vi "MOVE FRAME.vi"(8 "error in (no error)":errorcluster, 9 "return value":cluster{"x":dbl, "y":dbl}, 10 "Boolean":bool, 11 "Queue in":refnum<queue>) -> (0 "error out":errorcluster, 1 "Initial coordinates (m)":cluster{"Xc":sgl, "Yc":sgl} {"Yc" format="%.4p"; "Xc" format="%.4p"}, 2 "Final coordinates (m)":cluster{"Xc":sgl, "Yc":sgl} {"Yc" format="%.4p"; "Xc" format="%.4p"}, 3 "Queue out":refnum<queue>)   [LabVIEW 2025]
uses:
  Desktop/STM-Auto-Project/QMH CTLS/Scan_Params (QMH).ctl
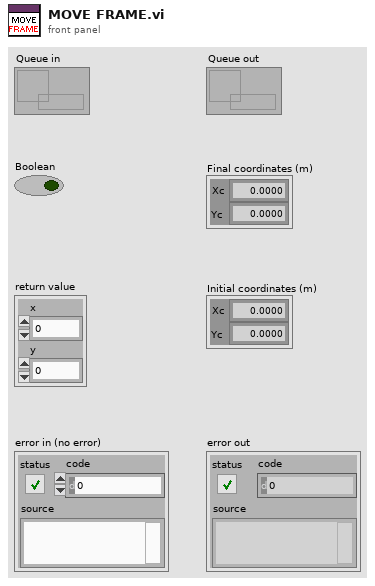
[diagram p1: front panel]
types:
  T1 = enum16{"1. BIAS", "2. INIT_SCAN", "3. SCAN_IDLE", "4. INTER_SCAN", "5. NEW_COORDS_&_FRAME", "6. FINAL_SCAN", "7. POLL BIAS ", "8. Z-CONT.", "9. STOP"}
  T2 = typedef "Scan_Params (QMH).ctl" = cluster{"Setpoint (I)":dbl[], "Bias (V)":dbl[], "Number of scans":u8, "Port number (3364)":u32, "Avoid zero threshold (V)":dbl, "Current State":enum16{"1. BIAS", "2. INIT_SCAN", "3. SCAN_IDLE", "4. INTER_SCAN", "5. NEW_COORDS_&_FRAME", "6. FINAL_SCAN", "7. POLL BIAS ", "8. Z-CONT.", "9. STOP"}}
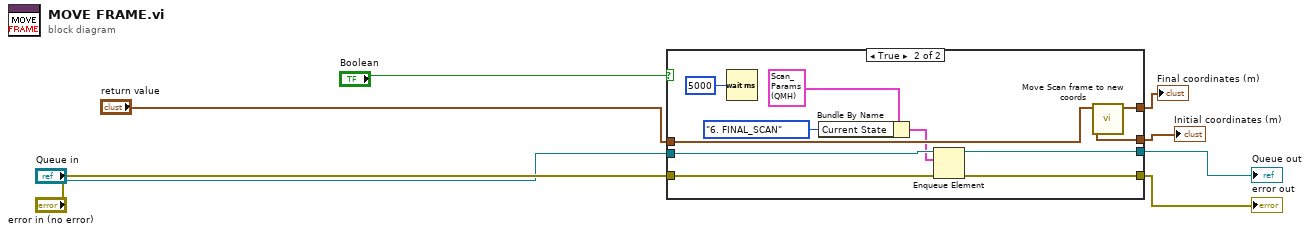
[diagram p0: block diagram]
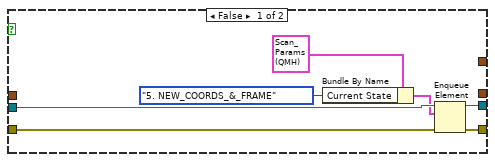
[diagram p2: hidden frame]
diagram:
  n1 = case shown="True" "Boolean" {
    tunnel: "return value" -> [_ w25]
    tunnel: "Queue in" -> [w15 w24]
    tunnel: [w14 w23] -> w3
    tunnel: [w12 w22] -> w4
    tunnel: "error in (no error)" -> [w13 w21]
    tunnel: [_ w19] -> w6
    tunnel: [_ w17] -> w7
    frame False {
      n2 = Bundle By Name(cluster=T2 {"Setpoint (I)"=[], "Bias (V)"=[], "Number of scans"=1, "Port number (3364)"=3364, "Avoid zero threshold (V)"=0.004999999888241291, "Current State"=enum."2. INIT_SCAN"} ("element"), "Current State"=T1."5. NEW_COORDS_&_FRAME") -> (w10:T2)
      n3 = Enqueue Element(queue=w15, element=w10, error in (no error)=w13) -> (queue out=w14:refnum<queue>, error out=w12:errorcluster)  [unwired: 1 in, 1 out]
    }
    frame True {
      n4 = Wait (ms)(milliseconds to wait=u32 5000) -> ()  [unwired: 1 out]
      n5 = Bundle By Name(cluster=T2 {"Setpoint (I)"=[], "Bias (V)"=[], "Number of scans"=1, "Port number (3364)"=3364, "Avoid zero threshold (V)"=0.004999999888241291, "Current State"=enum."2. INIT_SCAN"} ("element"), "Current State"=T1."6. FINAL_SCAN") -> (w18:T2)
      n6 = Enqueue Element(queue=w24, element=w18, error in (no error)=w21) -> (queue out=w23:refnum<queue>, error out=w22:errorcluster)  [unwired: 1 in, 1 out]
      n7 = call "Move Scan frame to new coords.vi"("Translation (m)"=w25) -> ("Final coordinates (m)"=w19:cluster{"Xc":sgl, "Yc":sgl}, "Initial coordinates (m)"=w17:cluster{"Xc":sgl, "Yc":sgl})  [unwired: 8 in, 1 out]
    }
  }
  "Final coordinates (m)" <- w6
  "Initial coordinates (m)" <- w7
  "error out" <- w4
  "Queue out" <- w3
